vi "MGI Rotate Vector (DBL).vi"(1 "Right Hand Rotation":dbl format="%.2f", 2 "Rotation Axis":T1, 3 "Input Vector":dbl[](array[numeric]) format="%.2f") -> (0 "Rotated Vector":dbl[](array[numeric]) format="%.2f")   [LabVIEW 2020]
doc: "Perform a 3D vector rotation about a coordinate axis.\n\nAuthored by David A. Moore\nsupport@mooregoodideas.com\nwww.mooregoodideas.com\n\nCopyright (c) 2010, Moore Good Ideas, Inc.\n\nAll rights reserved.\n\nRedistribution and use in source and binary forms, with or without modification, are permitted provided that the following conditions are met:\n\n * Redistributions of source code must retain the above copyright notice, this list of conditions and the following disclaimer.\n * Redistributions in binary form must reproduce the above copyright notice, this list of conditions and the following disclaimer in the documentation and/or other materials provided with the distribution.\n * Neither the name of Moore Good Ideas, Inc. nor the names of its contributors may be used to endorse or promote products derived from this software without specific prior written permission.\n\nTHIS SOFTWARE IS PROVIDED BY THE COPYRIGHT HOLDERS AND CONTRIBUTORS \"AS IS\" AND ANY EXPRESS OR IMPLIED WARRANTIES, INCLUDING, BUT NOT LIMITED TO, THE IMPLIED WARRANTIES OF MERCHANTABILITY AND FITNESS FOR A PARTICULAR PURPOSE ARE DISCLAIMED. IN NO EVENT SHALL THE COPYRIGHT OWNER OR CONTRIBUTORS BE LIABLE FOR ANY DIRECT, INDIRECT, INCIDENTAL, SPECIAL, EXEMPLARY, OR CONSEQUENTIAL DAMAGES (INCLUDING, BUT NOT LIMITED TO, PROCUREMENT OF SUBSTITUTE GOODS OR SERVICES; LOSS OF USE, DATA, OR PROFITS; OR BUSINESS INTERRUPTION) HOWEVER CAUSED AND ON ANY THEORY OF LIABILITY, WHETHER IN CONTRACT, STRICT LIABILITY, OR TORT (INCLUDING NEGLIGENCE OR OTHERWISE) ARISING IN ANY WAY OUT OF THE USE OF THIS SOFTWARE, EVEN IF ADVISED OF THE POSSIBILITY OF SUCH DAMAGE.."
uses:
  <userlib>/_MGI/Coordinates/MGI Coordinate Axis Enum.ctl
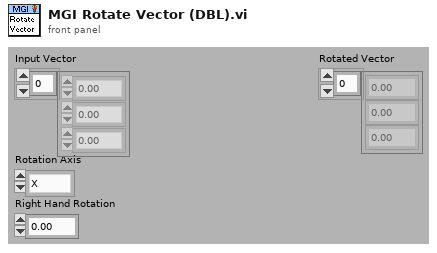
[diagram p1: front panel]
types:
  T1 = typedef "MGI Coordinate Axis Enum.ctl" = enum16{"X", "Y", "Z"}
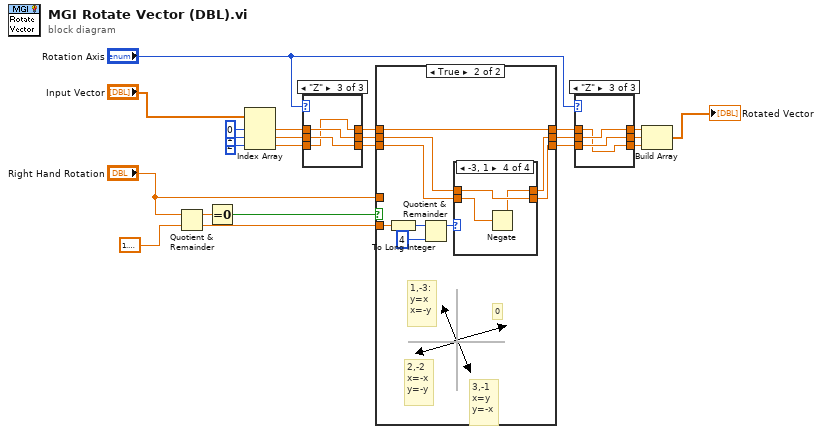
[diagram p0: block diagram]
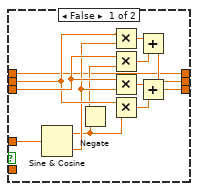
[diagram p2: hidden frame]
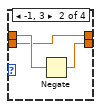
[diagram p4: hidden frame]
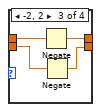
[diagram p5: hidden frame]
diagram:
  n1 = Quotient & Remainder(x="Right Hand Rotation", y=1.5707963267948966) -> (x-y*floor(x/y)=w23:dbl, floor(x/y)=w6:dbl)
  n2 = Equal To 0?(x=w23) -> (x = 0?=w7:bool)
  n3 = Index Array(array="Input Vector", index #1=0 ("Index"), index #2=1 ("Index"), index #3=2 ("Index")) -> (element #1=w19:dbl, element #2=w18:dbl, element #3=w17:dbl)
  n4 = case shown="\"Z\"" "Rotation Axis" {
    tunnel: [w26 w29 w30] -> w9
    tunnel: w19 -> [w26 w27 w31]
    tunnel: [w25 w28 w31] -> w10
    tunnel: w18 -> [w25 w29 w32]
    tunnel: [w24 w27 w32] -> w11
    tunnel: w17 -> [w24 w28 w30]
    frame "X" {
    }
    frame "Y" {
    }
    frame "Z" {
    }
  }
  n5 = case shown="True" w7 {
    tunnel: "Right Hand Rotation" -> [w45 _]
    tunnel: [w44 w46] -> w13
    tunnel: [w39 w47] -> w12
    tunnel: w11 -> [w38 w48]
    tunnel: w10 -> [w37 w49]
    tunnel: w9 -> [w33 w53]
    tunnel: [w33 w53] -> w8
    tunnel: w6 -> [_ w54]
    frame False {
      n6 = Sine & Cosine(0:w45) -> (1:w35:dbl, 2:w36:dbl)
      n7 = Negate(x=w35) -> (-x=w34:dbl)
      n8 = Multiply(x=w37, y=w36) -> (x*y=w40:dbl)
      n9 = Multiply(x=w38, y=w34) -> (x*y=w41:dbl)
      n10 = Multiply(x=w38, y=w36) -> (x*y=w43:dbl)
      n11 = Multiply(x=w37, y=w35) -> (x*y=w42:dbl)
      n12 = Add(x=w40, y=w41) -> (x+y=w39:dbl)
      n13 = Add(x=w43, y=w42) -> (x+y=w44:dbl)
    }
    frame True {
      # "3,-1\nx=y\ny=-x"
      # "2,-2\nx=-x\ny=-y"
      # "1,-3:\ny=x\nx=-y"
      # "0"
      n14 = To Long Integer(number=w54) -> (32bit integer=w52:i32)
      n15 = Quotient & Remainder(x=w52, y=4) -> (x-y*floor(x/y)=w50:i32)  [unwired: 1 out]
      n16 = case shown="-3, 1" w50 {
        tunnel: w49 -> [w56 w59 w63 w65]
        tunnel: w48 -> [w55 w57 w61 w66]
        tunnel: [w56 w57 w62 w64] -> w47
        tunnel: [w55 w58 w60 w65] -> w46
        frame ..-4, 0, 4.. {
        }
        frame -1, 3 {
          n17 = Negate(x=w59) -> (-x=w58:dbl)
        }
        frame -2, 2 {
          n18 = Negate(x=w63) -> (-x=w62:dbl)
          n19 = Negate(x=w61) -> (-x=w60:dbl)
        }
        frame -3, 1 {
          n20 = Negate(x=w66) -> (-x=w64:dbl)
        }
      }
    }
  }
  n21 = case shown="\"Z\"" "Rotation Axis" {
    tunnel: [w69 w70 w75] -> w16
    tunnel: w8 -> [w69 w71 w73]
    tunnel: [w68 w71 w74] -> w15
    tunnel: w12 -> [w68 w72 w75]
    tunnel: [w67 w72 w73] -> w14
    tunnel: w13 -> [w67 w70 w74]
    frame "X" {
    }
    frame "Y" {
    }
    frame "Z" {
    }
  }
  n22 = Build Array(w16, w15, w14) -> (→"Rotated Vector":dbl[])
